vi "enable_chop_acquisition - multi-channel with switch 2.vi"() -> ()   [LabVIEW 2019]
doc: "This example demonstrates how to enable the Chop feature in a continuously acquire buffered voltage measurement using a DAQmx device.\n\nFor instructions on how to connect your signals to the DAQ device, refer to your device documentation."
uses:
  <instrlib>/niSwitch/niSwitch.llb/niSwitch Topologies.ctl
  <instrlib>/niSwitch/niSwitch.llb/niSwitch Trigger Input.ctl
  <instrlib>/niSwitch/niSwitch.llb/niSwitch Scan Advanced Output.ctl
  <vilib>/DAQmx/read.llb/DAQmx Read (Analog 2D DBL NChan NSamp).vi
  <vilib>/DAQmx/create/channels.llb/DAQmx Create Channel (AI-Voltage-Basic).vi
  <vilib>/DAQmx/configure/timing.llb/DAQmx Timing (Sample Clock).vi
  <vilib>/DAQmx/miscellaneous.llb/DAQmx Fill In Error Info.vi
  <resource>/objmgr/daqmx.rc
panel:
  out "Measurement 4":dbl[](graph)
  out "Measurement 3":dbl[](graph)
  out "Measurement 2":dbl[](graph)
  out "error out":errorcluster
  in  "Total # of Channels":i32=37
  out "Elapsed Time (s)":dbl=1.576304575999984 format="%#_3g"
  in  "resource name":refnum<k15>="Switch" caption="Resource Name"
  in  "scan list":string="ch0->com0;" caption="Scan List"
  in  "topology name":T1="2530/2-Wire 64x1 Mux" caption="Topology Name"
  in  "Chop":bool=TRUE
  in  "Stop":bool
  out "Measurement":dbl[](graph)
  in  "Terminal Configuration":i32(ring)=10106 items=["default"=-1, "RSE"=10083, "NRSE"=10078, "Differential"=10106, "Pseudodifferential"=12529]
  in  "Max Voltage":dbl=10.0
  in  "Min Voltage":dbl=-10.0
  in  "Physical Channel":tag="4309/ai0:3"
  # "Switch Settings"
  # "DAQmx Settings"
  # "On (T)"
  # "Off (F)"
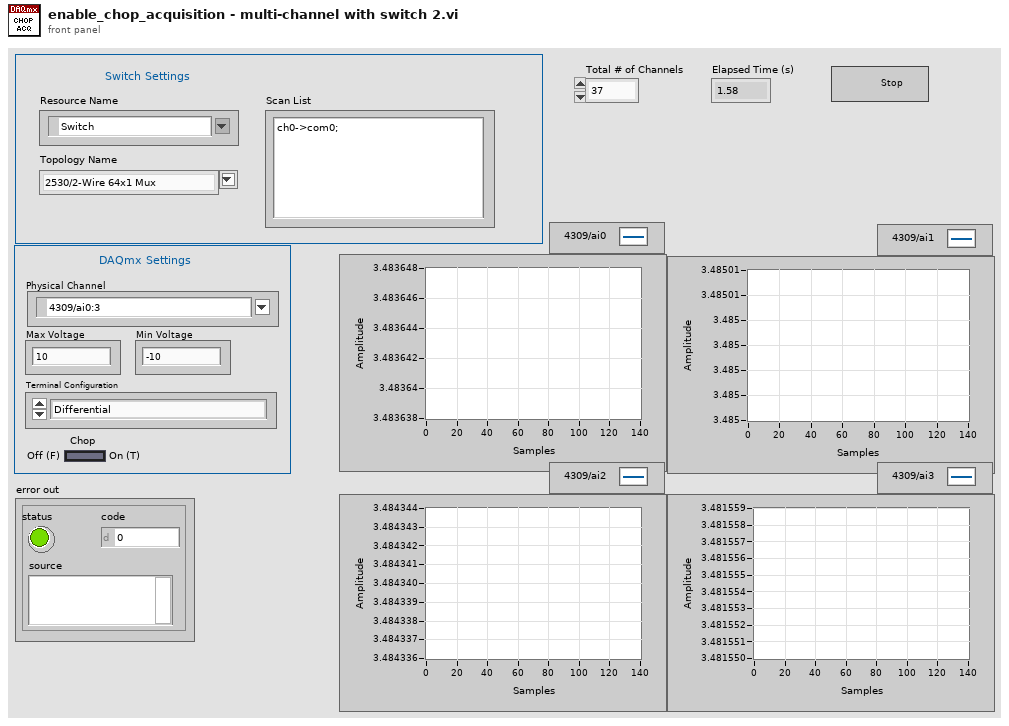
[diagram p1: front panel]
types:
  T1 = typedef "niSwitch Topologies.ctl" = string
  T2 = typedef "niSwitch Scan Advanced Output.ctl" = enum16{"None", "External", "TTL0", "TTL1", "TTL2", "TTL3", "TTL4", "TTL5", "TTL6", "TTL7", "ECL0", "ECL1", "PXI Star", "Rear Connector", "Front Connector", "Rear Connector Module 1", "Rear Connector Module 2", "Rear Connector Module 3", "Rear Connector Module 4", "Rear Connector Module 5", "Rear Connector Module 6", "Rear Connector Module 7", "Rear Connector Module 8", "Rear Connector Module 9", "Rear Connector Module 10", "Rear Connector Module 11", "Rear Connector Module 12", "Front Connector Module 1", "Front Connector Module 2", "Front Connector Module 3", "Front Connector Module 4", "Front Connector Module 5", "Front Connector Module 6", "Front Connector Module 7", "Front Connector Module 8", "Front Connector Module 9", "Front Connector Module 10", "Front Connector Module 11", "Front Connector Module 12"}
  T3 = typedef "niSwitch Trigger Input.ctl" = enum16{"Immediate", "External", "TTL0", "TTL1", "TTL2", "TTL3", "TTL4", "TTL5", "TTL6", "TTL7", "ECL0", "ECL1", "PXI Star", "Software Trigger Function", "Rear Connector", "Front Connector", "Rear Connector of Module 1", "Rear Connector of Module 2", "Rear Connector of Module 3", "Rear Connector of Module 4", "Rear Connector of Module 5", "Rear Connector of Module 6", "Rear Connector of Module 7", "Rear Connector of Module 8", "Rear Connector of Module 9", "Rear Connector of Module 10", "Rear Connector of Module 11", "Rear Connector of Module 12", "Front Connector of Module 1", "Front Connector of Module 2", "Front Connector of Module 3", "Front Connector of Module 4", "Front Connector of Module 5", "Front Connector of Module 6", "Front Connector of Module 7", "Front Connector of Module 8", "Front Connector of Module 9", "Front Connector of Module 10", "Front Connector of Module 11", "Front Connector of Module 12"}
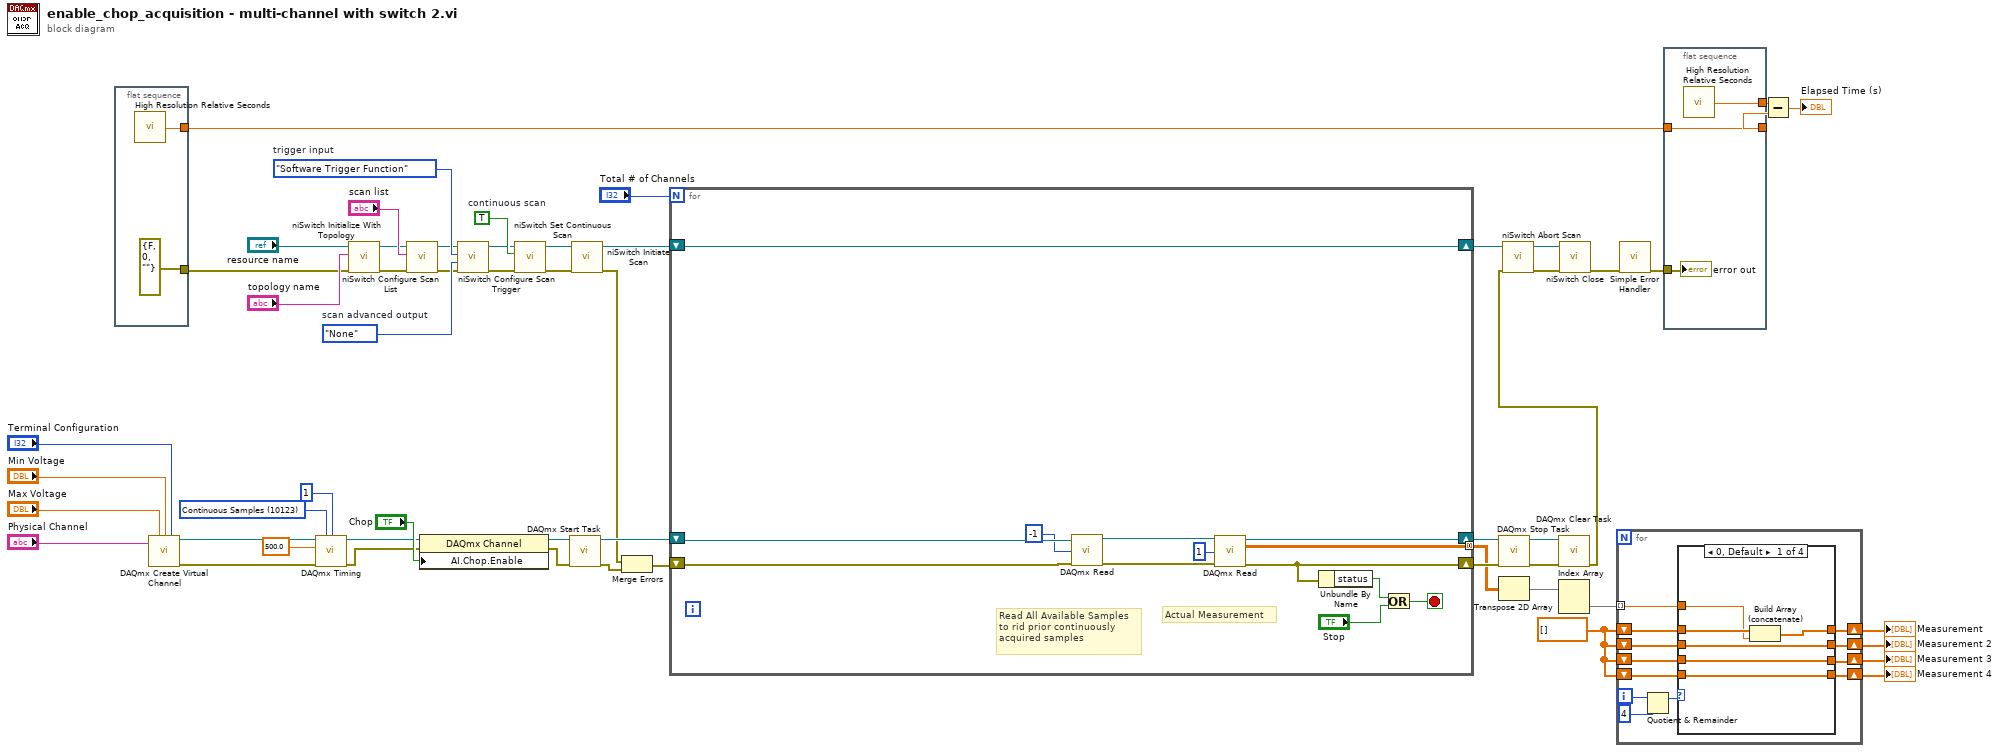
[diagram p0: block diagram]
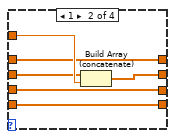
[diagram p2: hidden frame]
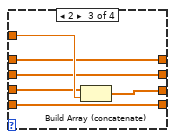
[diagram p3: hidden frame]
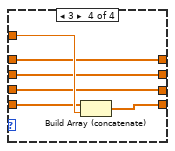
[diagram p4: hidden frame]
diagram:
  w4 = dbl[] [] ("History Data")
  w15 = 10123 items=["Finite Samples"=10178, "Continuous Samples"=10123, "Hardware Timed Single Point"=12522] ("sample mode")
  w49 = niSwitch_Scan_Advanced_Output."None"  # scan advanced output
  w48 = niSwitch_Trigger_Input."Software Trigger Function"  # trigger input
  w40 = TRUE  # continuous scan
  n1 = flat-sequence {
    tunnel: [w59] -> w28
    tunnel: [errorcluster {"status"=FALSE, "code"=0, "source"=""} ("error out")] -> w29
    frame #0 {
      n2 = call <vilib>:"High Resolution Relative Seconds.vi"() -> ("relative seconds"=w59:dbl)
    }
  }
  n3 = call-poly <vilib>:"DAQmx Create Virtual Channel.vi"("maximum value"="Max Voltage", "minimum value"="Min Voltage", "input terminal configuration"="Terminal Configuration", "physical channels"="Physical Channel") -> ("task out"=w21:refnum<k21>, "error out"=w24:errorcluster)  [unwired: 10 in]
  n4 = call-poly <vilib>:"DAQmx Timing.vi"("task/channels in"=w21, "sample mode"=w15, "samples per channel"=1, "rate"=500.0, "error in"=w24) -> ("task out"=w22:refnum<k21>, "error out"=w23:errorcluster)  [unwired: 9 in]
  n5 = call <instrlib>:"niSwitch Initialize With Topology.vi"("error in (no error)"=w29, "topology name"="topology name", "resource name"="resource name") -> ("error out"=w45:errorcluster, "instrument handle out"=w44:refnum<k15>)  [unwired: 2 in, 5 out]
  n6 = call <instrlib>:"niSwitch Configure Scan List.vi"("error in (no error)"=w45, "scan list"="scan list", "instrument handle"=w44) -> ("error out"=w38:errorcluster, "instrument handle out"=w36:refnum<k15>)  [unwired: 1 in, 6 out]
  n7 = property class="DAQmx Channel"(reference=w22, error in=w23, "AI.Chop.Enable"="Chop") -> (reference out=w20:refnum<k21>, error out=w19:errorcluster)
  n8 = call <instrlib>:"niSwitch Configure Scan Trigger.vi"("error in (no error)"=w38, "scan advanced output (External)"=w49, "trigger input (External)"=w48, "instrument handle"=w36) -> ("error out"=w39:errorcluster, "instrument handle out"=w35:refnum<k15>)  [unwired: 1 in, 5 out]
  n9 = call <instrlib>:"niSwitch Set Continuous Scan.vi"("error in (no error)"=w39, "continuous scan (False)"=w40, "instrument handle"=w35) -> ("error out"=w42:errorcluster, "instrument handle out"=w41:refnum<k15>)  [unwired: 7 out]
  n10 = call <vilib>:"DAQmx Start Task.vi"("task/channels in"=w20, "error in"=w19) -> ("task out"=w18:refnum<k21>, "error out"=w2:errorcluster)  [unwired: 12 in]
  n11 = call <instrlib>:"niSwitch Initiate Scan.vi"("error in (no error)"=w42, "instrument handle"=w41) -> ("error out"=w1:errorcluster, "instrument handle out"=w32:refnum<k15>)  [unwired: 8 out]
  n12 = Merge Errors(w1, w2) -> (w3:errorcluster)
  n13 = for {
    N: "Total # of Channels" -> [_]
    shift-right: [w60] -> w17
    shift-left: w32 -> [w60]
    shift-right: [w64] -> w13
    shift-left: w3 -> [w61]
    shift-right: [w63] -> w12
    shift-left: w18 -> [w70]
    tunnel: [w62] -> w11 mode=concatenating
    stop <- w71 stop-if-true
    # "Read All Available Samples\nto rid prior continuously\nacquired samples"
    # "Actual Measurement"
    n14 = call-poly <vilib>:"DAQmx Read.vi"("task/channels in"=w70, "number of samples per channel"=-1, "error in"=w61) -> ("task out"=w69:refnum<k21>, "error out"=w68:errorcluster)  [unwired: 10 in, 1 out]
    n15 = call-poly <vilib>:"DAQmx Read.vi"("task/channels in"=w69, "number of samples per channel"=1, "error in"=w68) -> ("task out"=w63:refnum<k21>, "data"=w62:dbl[][], "error out"=w64:errorcluster)  [unwired: 10 in]
    n16 = Unbundle By Name(w64) -> ("status"=w65:bool)
    n17 = Or(x=w65, y="Stop") -> (x .or. y?=w71:bool)
  }
  n18 = call <vilib>:"DAQmx Stop Task.vi"("task/channels in"=w12, "error in"=w13) -> ("task out"=w52:refnum<k21>, "error out"=w53:errorcluster)  [unwired: 12 in]
  n19 = Transpose 2D Array(2D array=w11) -> (transposed array=w10:dbl[][])
  n20 = call <vilib>:"DAQmx Clear Task.vi"("task in"=w52, "error in"=w53) -> ("error out"=w34:errorcluster)  [unwired: 13 in]
  n21 = call <instrlib>:"niSwitch Abort Scan.vi"("error in (no error)"=w34, "instrument handle"=w17) -> ("error out"=w43:errorcluster, "instrument handle out"=w37:refnum<k15>)  [unwired: 8 out]
  n22 = Index Array(array=w10) -> (element=w9:dbl[])  [unwired: 2 in]
  n23 = call <instrlib>:"niSwitch Close.vi"("error in (no error)"=w43, "instrument handle"=w37) -> ("error out"=w33:errorcluster)  [unwired: 9 out]
  n24 = for {
    tunnel: w9 -> [w81] mode=indexing
    shift-right: [w79] -> w8
    shift-left: w4 -> [w80]
    shift-right: [w78] -> w7
    shift-left: w4 -> [w77]
    shift-right: [w76] -> w6
    shift-left: w4 -> [w75]
    shift-right: [w74] -> w5
    shift-left: w4 -> [w73]
    i -> [w84]
    n25 = Quotient & Remainder(x=w84, y=4) -> (x-y*floor(x/y)=w82:i32)  [unwired: 1 out]
    n26 = case shown="0, Default" w82 {
      tunnel: w81 -> [w88 w96 w102 w108]
      tunnel: w80 -> [w89 w93 w99 w105]
      tunnel: [w90 w93 w99 w105] -> w79
      tunnel: [w87 w95 w98 w104] -> w78
      tunnel: w77 -> [w87 w94 w98 w104]
      tunnel: [w86 w92 w101 w103] -> w76
      tunnel: w75 -> [w86 w92 w100 w103]
      tunnel: [w85 w91 w97 w107] -> w74
      tunnel: w73 -> [w85 w91 w97 w106]
      frame 0, Default {
        n27 = Build Array (concatenate)(w89, w88) -> (w90:dbl[])
      }
      frame 1 {
        n28 = Build Array (concatenate)(w94, w96) -> (w95:dbl[])
      }
      frame 2 {
        n29 = Build Array (concatenate)(w100, w102) -> (w101:dbl[])
      }
      frame 3 {
        n30 = Build Array (concatenate)(w106, w108) -> (w107:dbl[])
      }
    }
  }
  "Measurement" <- w8
  "Measurement 2" <- w7
  "Measurement 3" <- w6
  "Measurement 4" <- w5
  n31 = call <vilib>:"Simple Error Handler.vi"("error in (no error)"=w33) -> ("error out"=w30:errorcluster)  [unwired: 1 in, 7 out]
  n32 = flat-sequence {
    tunnel: w30 -> [w109]
    tunnel: [w111] -> w27
    tunnel: w28 -> [w110]
    tunnel: [w110] -> w26
    frame #0 {
      n33 = call <vilib>:"High Resolution Relative Seconds.vi"() -> ("relative seconds"=w111:dbl)
      "error out" <- w109
    }
  }
  n34 = Subtract(x=w27, y=w26) -> (x-y=→"Elapsed Time (s)":dbl)
